vi "UI FGV.vi"(1 "Data in":T1={"Oscillator"={"Waveform Type"=0, "Pulse Width"=0.0, "Sub oscillator"=enum."Off", "Frequency"=0.0, "Amplitude"=0.0}, "ADSR"={"A"=0, "D"=0, "S"=0, "R"=0, "Volume"=0.0}, "Lowpass filter"={"On / Off"=FALSE, "Cutoff"=20.0}, "Tremolo"={"Rate"=0.0, "Frequency"=20.0, " on/off "=FALSE}, "Play sound"=FALSE} {"Tremolo"."Frequency" min=0.0 max=25.0 scale=0.0..25.0; "Tremolo"."Rate" min=0.0 max=1.0 scale=0.0..1.0; "Lowpass filter"."Cutoff" min=20.0 max=20000.0 scale=20.0..20000.0; "ADSR"."Volume" min=0.0 max=100.0 scale=0.0..100.0; "ADSR"."R" scale=0.0..100.0; "ADSR"."S" scale=0.0..100.0; "ADSR"."D" scale=0.0..100.0; "ADSR"."A" scale=0.0..100.0; "Oscillator"."Amplitude" scale=0.0..10.0; "Oscillator"."Frequency" scale=20.0..20000.0; "Oscillator"."Pulse Width" min=0.0 max=100.0 scale=0.0..100.0; "Oscillator"."Waveform Type" items=["Sine Wave", "Triangle Wave", "Square Wave", "Sawtooth Wave"]}, 2 "Mode":T7) -> (0 "Data out":T1={"Oscillator"={"Waveform Type"=0, "Pulse Width"=0.0, "Sub oscillator"=enum."Off", "Frequency"=0.0, "Amplitude"=0.0}, "ADSR"={"A"=0, "D"=0, "S"=0, "R"=0, "Volume"=0.0}, "Lowpass filter"={"On / Off"=FALSE, "Cutoff"=20.0}, "Tremolo"={"Rate"=0.0, "Frequency"=20.0, " on/off "=FALSE}, "Play sound"=FALSE} {"Tremolo"."Frequency" min=0.0 max=25.0 scale=0.0..25.0; "Tremolo"."Rate" min=0.0 max=1.0 scale=0.0..1.0; "Lowpass filter"."Cutoff" min=20.0 max=20000.0 scale=20.0..20000.0; "ADSR"."Volume" min=0.0 max=100.0 scale=0.0..100.0; "ADSR"."R" scale=0.0..100.0; "ADSR"."S" scale=0.0..100.0; "ADSR"."D" scale=0.0..100.0; "ADSR"."A" scale=0.0..100.0; "Oscillator"."Amplitude" scale=0.0..10.0; "Oscillator"."Frequency" scale=20.0..20000.0; "Oscillator"."Pulse Width" min=0.0 max=100.0 scale=0.0..100.0; "Oscillator"."Waveform Type" items=["Sine Wave", "Triangle Wave", "Square Wave", "Sawtooth Wave"]})   [LabVIEW 2019]
uses:
  Type Definitions/UI.ctl
  Type Definitions/UIOscillatorParam.ctl
  Type Definitions/Sub Oscillalator Type.ctl
  Type Definitions/UIADSRParam.ctl
  Type Definitions/UILowpassParam.ctl
  Type Definitions/UITremolo.ctl
  Type Definitions/DataInOut.ctl
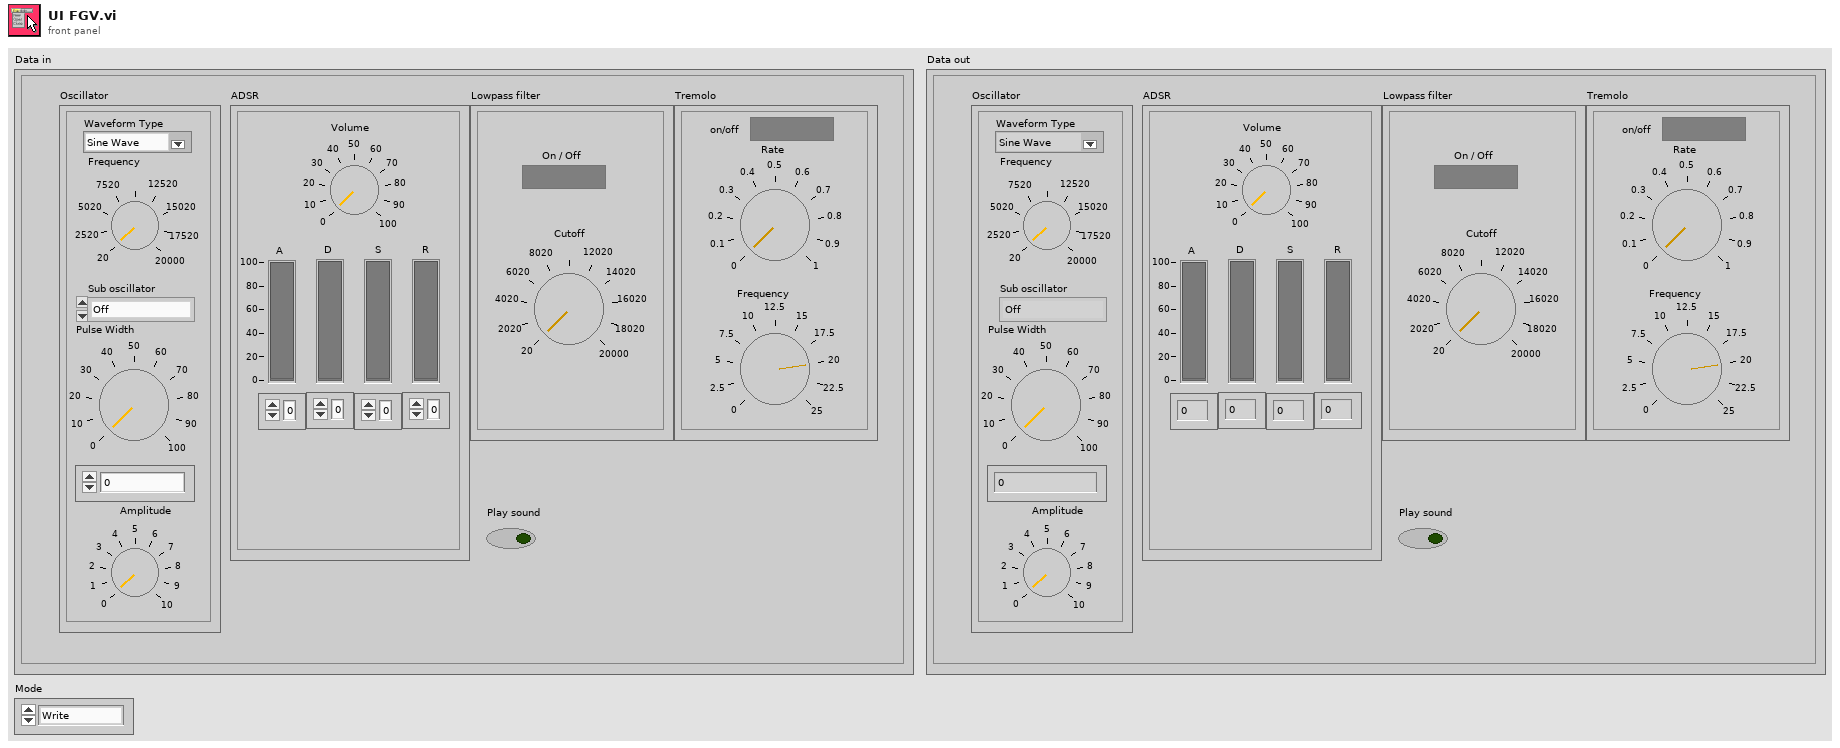
[diagram p1: front panel]
types:
  T1 = typedef "UI.ctl" = cluster{"Oscillator":T2, "ADSR":T4, "Lowpass filter":T5, "Tremolo":T6, "Play sound":bool}
  T2 = typedef "UIOscillatorParam.ctl" = cluster{"Waveform Type":u16, "Pulse Width":dbl, "Sub oscillator":T3, "Frequency":dbl, "Amplitude":dbl}
  T3 = typedef "Sub Oscillalator Type.ctl" = enum16{"Off", "One Octave", "Two Octaves"}
  T4 = typedef "UIADSRParam.ctl" = cluster{"A":i32, "D":i32, "S":i32, "R":i32, "Volume":dbl}
  T5 = typedef "UILowpassParam.ctl" = cluster{"On / Off":bool, "Cutoff":dbl}
  T6 = typedef "UITremolo.ctl" = cluster{"Rate":dbl, "Frequency":dbl, " on/off ":bool}
  T7 = typedef "DataInOut.ctl" = enum16{"Write", "Read"}
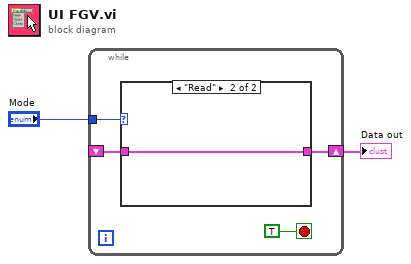
[diagram p0: block diagram]
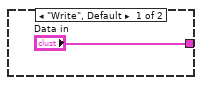
[diagram p2: hidden frame]
diagram:
  n1 = while {
    tunnel: "Mode" -> [w5]
    shift-right: [w4] -> w1
    shift-left: _ -> [w3]
    stop <- TRUE stop-if-true
    n2 = case shown="\"Read\"" w5 {
      tunnel: ["Data in" w8] -> w4
      tunnel: w3 -> [_ w8]
      frame "Write", Default {
      }
      frame "Read" {
      }
    }
  }
  "Data out" <- w1
